vi "FICHEROS.vi"() -> ()   [LabVIEW 2020]
panel:
  in  "error in":errorcluster
  in  "Direccion":path
  in  "Nombre Fichero":string
  in  "Combo Box":string(combo)
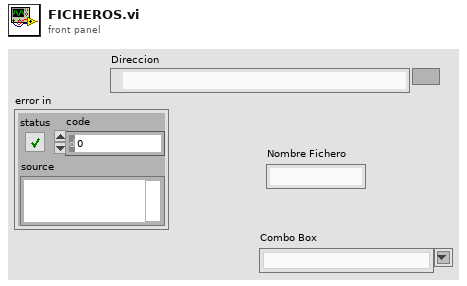
[diagram p1: front panel]
types:
  T1 = enum16{"open", "replace", "create", "open or create", "replace or create", "replace or create with confirmation"}
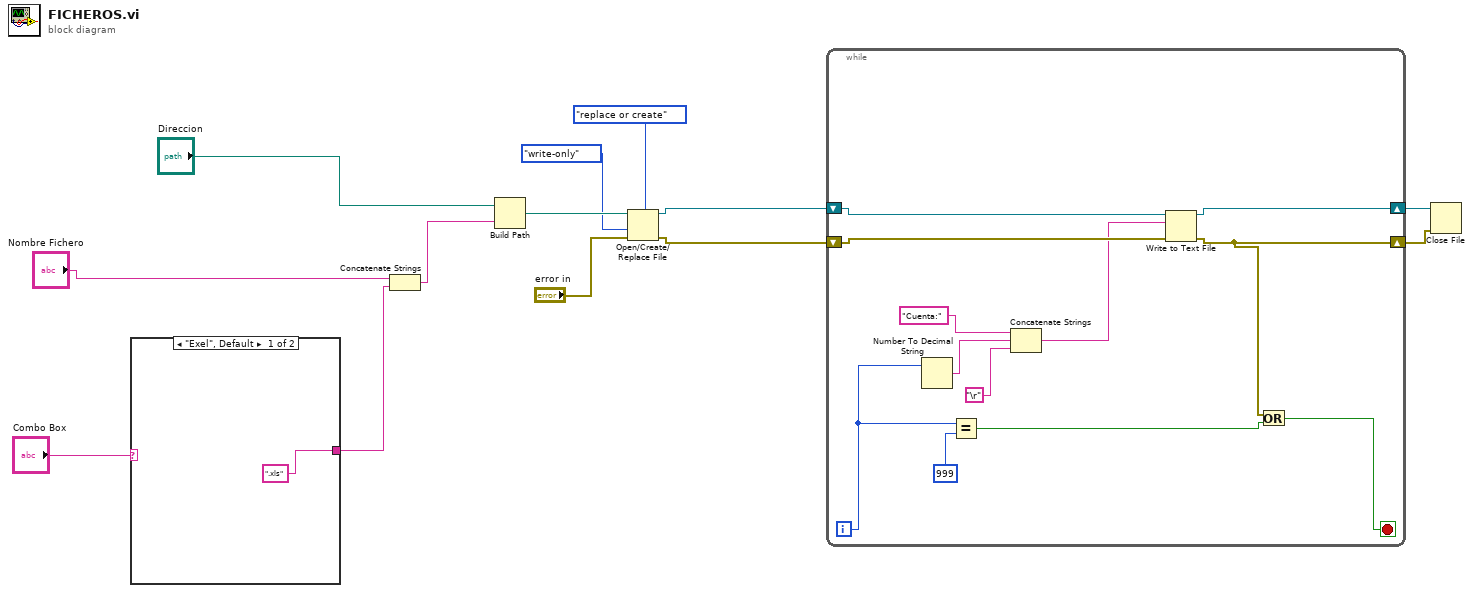
[diagram p0: block diagram]
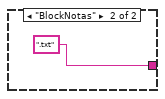
[diagram p2: hidden frame]
diagram:
  n1 = case shown="\"Exel\", Default" "Combo Box" {
    tunnel: [".xls" ".txt"] -> w11
    frame "Exel", Default {
    }
    frame "BlockNotas" {
    }
  }
  n2 = Concatenate Strings("Nombre Fichero", w11) -> (w10:string)
  n3 = Build Path(base path="Direccion", name or relative path=w10) -> (appended path=w8:path)
  n4 = Open/Create/Replace File(file path (use dialog)=w8, error in="error in", operation (0:open)=T1."replace or create", access (0:read/write)=enum16{"read/write", "read-only", "write-only"}."write-only") -> (refnum out=w4:refnum<file>, error out=w3:errorcluster)  [unwired: 2 in, 1 out]
  n5 = while {
    shift-right: [w23] -> w2
    shift-left: w4 -> [w24]
    shift-right: [w18] -> w1
    shift-left: w3 -> [w22]
    i -> [w20]
    stop <- w16 stop-if-true
    n6 = Number To Decimal String(number=w20) -> (decimal integer string=w26:string)  [unwired: 1 in]
    n7 = Equal?(x=w20, y=999) -> (x = y?=w17:bool)
    n8 = Concatenate Strings("Cuenta:", w26, "\r") -> (w21:string)
    n9 = Write to Text File(file (use dialog)=w24, text=w21, error in=w22) -> (refnum out=w23:refnum<file>, error out=w18:errorcluster)  [unwired: 1 in, 1 out]
    n10 = Or(x=w18, y=w17) -> (x .or. y?=w16:bool)
  }
  n11 = Close File(refnum=w2, error in=w1) -> ()  [unwired: 2 out]
